vi "Publish Sample.vi"(8 "error in (no error)":errorcluster, 9 "Sample":refnum<class "Sample.lvclass">, 11 "Capillary Line in":refnum<class "Capillary Line.lvclass">) -> (0 "error out":errorcluster, 3 "Capillary Line in 2":refnum<class "Capillary Line.lvclass">)   [LabVIEW 2015, in "cRIO-Carbondioxide.lvlib" / "CO2-Actor.lvlib" / "Capillary Line.lvclass"]
uses:
  Capillary Line.lvclass
  subs/Sample/Sample.lvclass
  Capillary Line.lvclass/Capillary Line.ctl
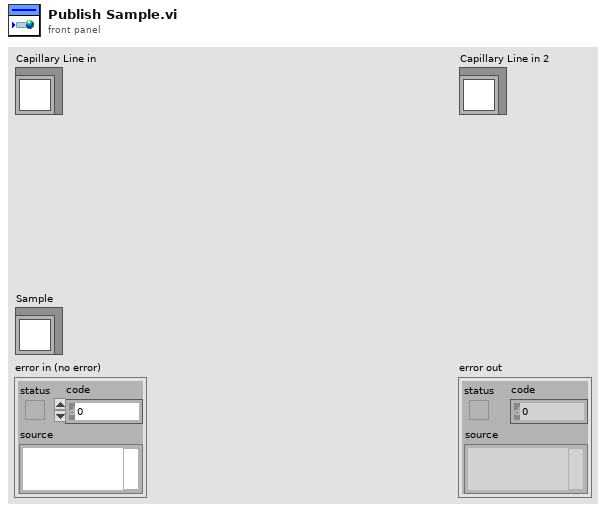
[diagram p1: front panel]
types:
  T1 = typedef "Sample Container.ctl" = cluster{"Sample In":refnum<k21>, "Sample Name":refnum<k21>, "Ti Cathode":refnum<k21>, "SampleQ":refnum<queue>}
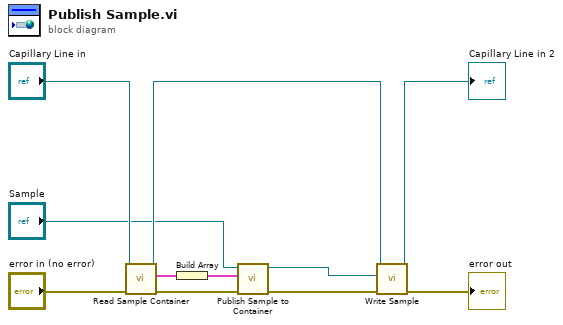
[diagram p0: block diagram]
diagram:
  n1 = call "Read Sample Container.vi"("error in (no error)"="error in (no error)", "Capillary Line in"="Capillary Line in") -> ("error out"=w6:errorcluster, "Container"=w5:T1, "Capillary Line out"=w8:refnum<class "Capillary Line.lvclass">)  [unwired: 6 in, 1 out]
  n2 = Build Array(w5) -> (w4:T1[])
  n3 = call "Publish Sample to Container.vi"("error in (no error)"=w6, "Containers"=w4, "Sample in"="Sample") -> ("error out"=w3:errorcluster, "Sample out"=w1:refnum<class "Sample.lvclass">)  [unwired: 7 in]
  n4 = call "Write Sample.vi"("error in (no error)"=w3, "Sample.lvclass"=w1, "Capillary Line in"=w8) -> ("error out"=→"error out":errorcluster, "Capillary Line out"=→"Capillary Line in 2":refnum<class "Capillary Line.lvclass">)  [unwired: 7 in]
